vi "Query Data Queue Storage Status.vi"(8 "error in (no error)":errorcluster, 11 "VISA resource name":refnum<visa-resource-name>) -> (0 "error out":errorcluster, 1 "Queue Capacity":i32, 2 "Item Count":i32, 3 "VISA resource name out":refnum<visa-resource-name>)   [LabVIEW 2015, in "Keithley 2600 Series.lvlib"]
doc: "Returns the data queue length and the items number."
uses:
  Keithley 2600 Series.lvlib
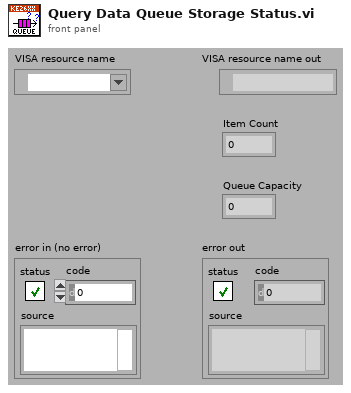
[diagram p1: front panel]
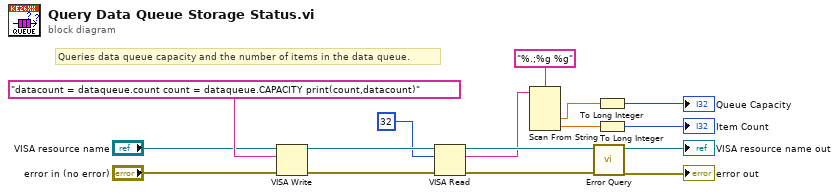
[diagram p0: block diagram]
diagram:
  # "Queries data queue capacity and the number of items in the data queue."
  n1 = VISA Write(VISA resource name="VISA resource name", write buffer="datacount = dataqueue.count count = dataqueue.CAPACITY print(count,datacount)", error in (no error)="error in (no error)") -> (VISA resource name out=w11:refnum<visa-resource-name>, error out=w10:errorcluster)  [unwired: 1 out]
  n2 = VISA Read(VISA resource name=w11, byte count=u32 32, error in (no error)=w10) -> (VISA resource name out=w8:refnum<visa-resource-name>, read buffer=w6:string, error out=w7:errorcluster)  [unwired: 1 out]
  n3 = Scan From String(format string="%.;%g %g", input string=w6) -> (output 1=w1:dbl, output 2=w2:dbl)  [unwired: 4 in, 3 out]
  n4 = call "Error Query.vi"("error in (no error)"=w7, "VISA resource name"=w8) -> ("error out"=→"error out":errorcluster, "VISA resource name out"=→"VISA resource name out":refnum<visa-resource-name>)  [unwired: 6 in, 2 out]
  n5 = To Long Integer(number=w1) -> (32bit integer=→"Queue Capacity":i32)
  n6 = To Long Integer(number=w2) -> (32bit integer=→"Item Count":i32)
